vi "dfd_FIR Spectral Factorization Scaling.vi"(9 "maximum phase in":dbl[](array[numeric]), 10 "minimum phase in":dbl[](array[numeric])) -> (1 "maximum phase":dbl[](array[numeric]), 2 "minimum phase":dbl[](array[numeric]))   [LabVIEW 2017, in "NI_DigFilter_FilterBank.lvlib"]
uses:
  <vilib>/addons/Digital Filter Design/NI_DigFilter_FilterBank.lvlib
  <vilib>/Analysis/baseanly.llb/Real Dot Product.vi
  <vilib>/Analysis/NI_AALBase.lvlib
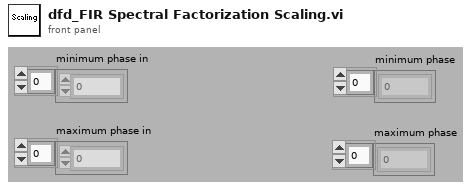
[diagram p1: front panel]
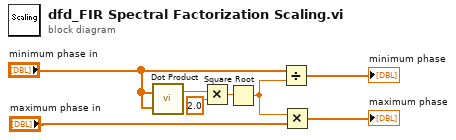
[diagram p0: block diagram]
diagram:
  n1 = call-poly <vilib>:"Dot Product.vi"("Y Vector"="minimum phase in", "X Vector"="minimum phase in") -> ("X * Y"=w8:dbl)  [unwired: 1 out]
  n2 = Multiply(x=w8, y=2.0) -> (x*y=w6:dbl)
  n3 = Square Root(x=w6) -> (sqrt(x)=w2:dbl)
  n4 = Divide(x="minimum phase in", y=w2) -> (x/y=→"minimum phase":dbl[])
  n5 = Multiply(x=w2, y="maximum phase in") -> (x*y=→"maximum phase":dbl[])
